vi "BundleMagic INI path.vi"() -> (3 "appended path":path)   [LabVIEW 2023]
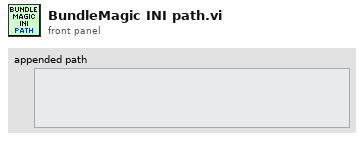
[diagram p1: front panel]
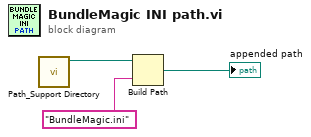
[diagram p0: block diagram]
diagram:
  n1 = call "Path_Support Directory.vi"() -> ("Support Directory"=w3:path)  [unwired: 11 in]
  n2 = Build Path(base path=w3, name or relative path="BundleMagic.ini") -> (appended path=→"appended path":path)
